vi "NI VeriStand - Send Packet to Host.vi"(10 "Element":u64, 11 "Prev":bool) -> (0 "Next":bool)   [LabVIEW 2020, in "NI_VS FPGA Support.lvlib"]
uses:
  <vilib>/NI VeriStand/FPGA/NI_VS FPGA Support.lvlib
  <vilib>/rvi/DataTransferAndStorage/Container/XNode/niFpgaContainer.xnode
  <vilib>/rvi/interface/RandomDataEmulation/nirviRandomDataFpgaReadWriteTemplate.vi
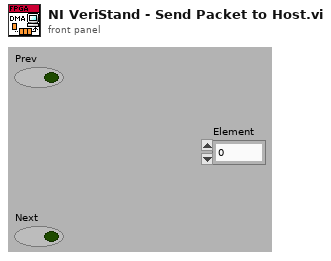
[diagram p1: front panel]
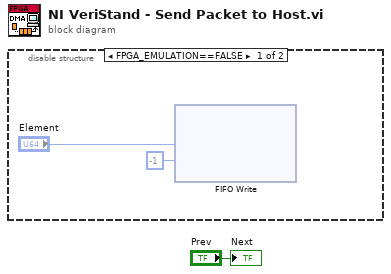
[diagram p0: block diagram]
diagram:
  n1 = disable-structure shown="FPGA_EMULATION==FALSE" {
    frame condition #0 {
      n2 = xnode ("FIFO Write")("Element"="Element", "Timeout"=-1) -> ()  [unwired: 1 in, 2 out]
    }
    frame condition #1 (active) {
    }
  }
  "Next" <- "Prev"
